vi "GetDigitalPosition.vi"(0 "Handle":u64, 1 "Controller Channel":i64) -> (7 "FT_Status":u64(ring) items=["FT_OK", "FT_INVALID_HANDLE", "FT_DEVICE_NOT_FOUND", "FT_DEVICE_NOT_OPENED", "FT_IO_ERROR", "FT_INSUFFICIENT_RESOURCES", "FT_INVALID_PARAMETER", "FT_INVALID_BAUD_RATE", "FT_DEVICE_NOT_OPENED_FOR_ERASE", "FT_DEVICE_NOT_OPENED_FOR_WRITE", "FT_FAILED_TO_WRITE_DEVICE", "FT_EEPROM_READ_FAILED", "FT_EEPROM_WRITE_FAILED", "FT_EEPROM_ERASE_FAILED", "FT_EEPROM_NOT_PRESENT", "FT_EEPROM_NOT_PROGRAMMED", "FT_INVALID_ARGS", "FT_NOT_SUPPORTED", "FT_OTHER_ERROR"], 9 "Position":i64)   [LabVIEW 2018]
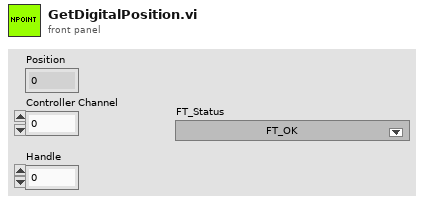
[diagram p1: front panel]
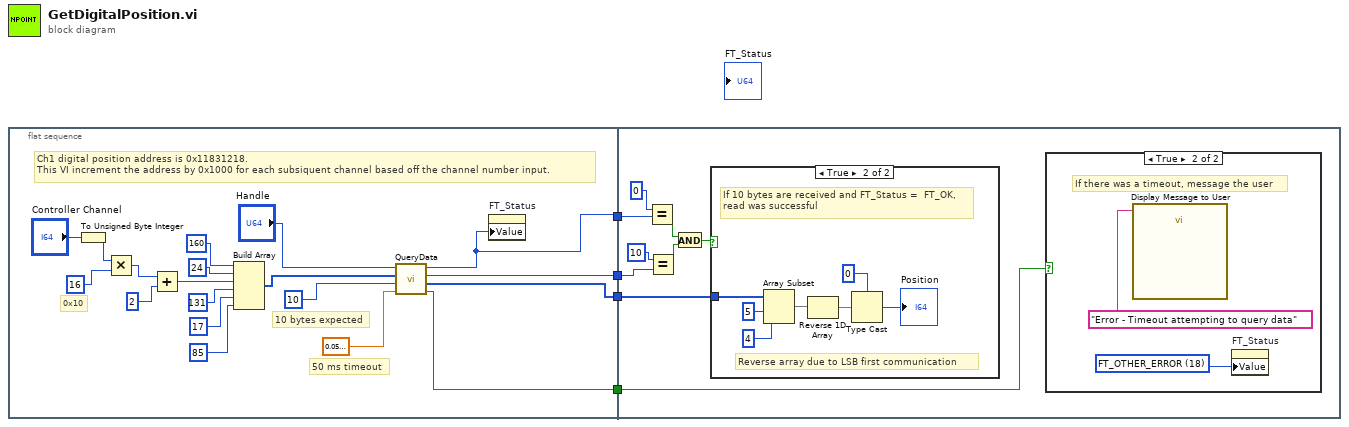
[diagram p0: block diagram]
diagram:
  n1 = flat-sequence {
    tunnel: [w9] -> w4
    tunnel: [w8] -> w3
    tunnel: [w7] -> w2
    tunnel: [w6] -> w1
    tunnel: w4 -> [w32]
    tunnel: w3 -> [w30]
    tunnel: w2 -> [w29]
    tunnel: w1 -> [w27]
    frame #0 {
      # "10 bytes expected"
      # "50 ms timeout"
      # "Ch1 digital position address is 0x11831218.\nThis VI increment the address by 0x1000 for each subsiquent channel based off the channel number input."
      # "0x10"
      n2 = To Unsigned Byte Integer(number="Controller Channel") -> (unsigned 8bit integer=w5:u8)
      n3 = Multiply(x=w5, y=u8 16) -> (x*y=w16:u8)
      n4 = Add(x=w16, y=u8 2 ("element")) -> (x+y=w15:u8)
      n5 = Build Array(u8 160 ("element"), u8 24 ("element"), w15, u8 131 ("element"), u8 17 ("element"), u8 85 ("element")) -> (w12:u8[])
      n6 = call "QueryData.vi"("TimeoutLengthSeconds"=sgl 0.05, "NumBytesExpected"=u64 10, "Message"=w12, "Handle"="Handle") -> ("Timeout"=w7:bool, "Return Array"=w8:u8[], "Bytes Read"=w9:u64, "FT_Status"=w6:u64)  [unwired: 4 in]
      n7 = property on="FT_Status" class="Ring (strict)"("Value"=w6) -> ()  [unwired: 2 in, 2 out]
    }
    frame #1 {
      n8 = Equal?(x=u64 0, y=w27) -> (x = y?=w25:bool)
      n9 = Equal?(x=u64 10, y=w32) -> (x = y?=w26:bool)
      n10 = And(x=w25, y=w26) -> (x .and. y?=w24:bool)
      n11 = case shown="True" w24 {
        tunnel: w30 -> [_ w41]
        frame False {
        }
        frame True {
          # "Reverse array due to LSB first communication"
          # "If 10 bytes are received and FT_Status =  FT_OK,\nread was successful"
          n12 = Array Subset(array=w41, index=5, length=4) -> (w37:u8[])
          n13 = Reverse 1D Array(array=w37) -> (reversed array=w36:u8[])
          n14 = Type Cast(type=0, x=w36) -> (*(type *) &x=→"Position":i32)
        }
      }
      n15 = case shown="True" w29 {
        frame False {
        }
        frame True {
          w33 = u64 18 items=["FT_OK", "FT_INVALID_HANDLE", "FT_DEVICE_NOT_FOUND", "FT_DEVICE_NOT_OPENED", "FT_IO_ERROR", "FT_INSUFFICIENT_RESOURCES", "FT_INVALID_PARAMETER", "FT_INVALID_BAUD_RATE", "FT_DEVICE_NOT_OPENED_FOR_ERASE", "FT_DEVICE_NOT_OPENED_FOR_WRITE", "FT_FAILED_TO_WRITE_DEVICE", "FT_EEPROM_READ_FAILED", "FT_EEPROM_WRITE_FAILED", "FT_EEPROM_ERASE_FAILED", "FT_EEPROM_NOT_PRESENT", "FT_EEPROM_NOT_PROGRAMMED", "FT_INVALID_ARGS", "FT_NOT_SUPPORTED", "FT_OTHER_ERROR"] ("FT_Status")
          # "If there was a timeout, message the user"
          n16 = call "Display Message to User"("Message"="Error - Timeout attempting to query data") -> ()  [unwired: 9 in, 2 out]
          n17 = property on="FT_Status" class="Ring (strict)"("Value"=w33) -> ()  [unwired: 2 in, 2 out]
        }
      }
    }
  }
